vi "Front Grabber Control Read.vi"(1 "Controller State":T1 {"POV" items=["None"=-1, "POV Up"=0, "POV Up Right"=1, "POV Right"=2, "POV Down Right"=3, "POV Down"=4, "POV Down Left"=5, "POV Left"=6, "POV Up Left"=7]}) -> (0 "State out":i16)   [LabVIEW 2010]
uses:
  <vilib>/FTC/FTC ControllerState.ctl
  <vilib>/FTC/FTC POVState.ctl
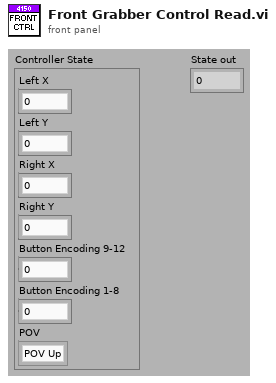
[diagram p1: front panel]
types:
  T1 = typedef "FTC ControllerState.ctl" = cluster{"Left X":i8, "Left Y":i8, "Right X":i8, "Right Y":i8, "Button Encoding 9-12":u8, "Button Encoding 1-8":u8, "POV":T2}
  T2 = typedef "FTC POVState.ctl" = i8
  T3 = typedef "FTC ButtonState.ctl" = cluster{"Button 1":bool, "Button 2":bool, "Button 3":bool, "Button 4":bool, "Button 5":bool, "Button 6":bool, "Button 7":bool, "Button 8":bool, "Button 9":bool, "Button 10":bool, "Button 11":bool, "Button 12":bool, "POV":T2}
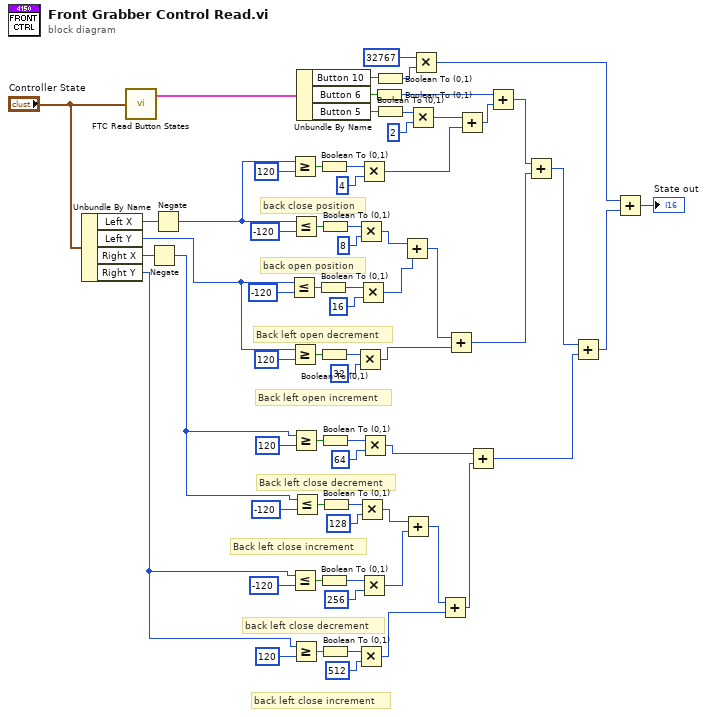
[diagram p0: block diagram]
diagram:
  # "Back left open increment"
  # "Back left open decrement"
  # "back open position"
  # "back left close decrement"
  # "Back left close decrement"
  # "Back left close increment"
  # "back left close increment"
  # "back close position"
  n1 = Unbundle By Name("Controller State") -> ("Left X"=w50:i8, "Left Y"=w40:i8, "Right X"=w14:i8, "Right Y"=w13:i8)
  n2 = call <vilib>:"FTC Read Button States.vi"("Controller State"="Controller State") -> ("Button States"=w53:T3)  [unwired: 2 in, 1 out]
  n3 = Negate(x=w14) -> (-x=w7:i8)
  n4 = Negate(x=w50) -> (-x=w8:i8)
  n5 = Less Or Equal?(x=w40, y=i8 -120) -> (x <= y?=w43:bool)
  n6 = Greater Or Equal?(x=w8, y=i8 120) -> (x >= y?=w55:bool)
  n7 = Greater Or Equal?(x=w40, y=i8 120) -> (x >= y?=w44:bool)
  n8 = Less Or Equal?(x=w13, y=i8 -120) -> (x <= y?=w28:bool)
  n9 = Less Or Equal?(x=w8, y=i8 -120) -> (x <= y?=w56:bool)
  n10 = Greater Or Equal?(x=w7, y=i8 120) -> (x >= y?=w20:bool)
  n11 = Greater Or Equal?(x=w13, y=i8 120) -> (x >= y?=w27:bool)
  n12 = Less Or Equal?(x=w7, y=i8 -120) -> (x <= y?=w19:bool)
  n13 = Unbundle By Name(w53) -> ("Button 10"=w6:bool, "Button 6"=w54:bool, "Button 5"=w63:bool)
  n14 = Boolean To (0,1)(Boolean=w43) -> (0, 1=w45:i16)
  n15 = Boolean To (0,1)(Boolean=w55) -> (0, 1=w57:i16)
  n16 = Boolean To (0,1)(Boolean=w44) -> (0, 1=w47:i16)
  n17 = Boolean To (0,1)(Boolean=w28) -> (0, 1=w26:i16)
  n18 = Boolean To (0,1)(Boolean=w56) -> (0, 1=w61:i16)
  n19 = Boolean To (0,1)(Boolean=w20) -> (0, 1=w18:i16)
  n20 = Boolean To (0,1)(Boolean=w27) -> (0, 1=w24:i16)
  n21 = Boolean To (0,1)(Boolean=w19) -> (0, 1=w16:i16)
  n22 = Multiply(x=w47, y=i16 32) -> (x*y=w36:i16)
  n23 = Multiply(x=w61, y=i16 8) -> (x*y=w39:i16)
  n24 = Multiply(x=w24, y=i16 512) -> (x*y=w34:i16)
  n25 = Multiply(x=w16, y=i16 128) -> (x*y=w31:i16)
  n26 = Multiply(x=w45, y=i16 16) -> (x*y=w38:i16)
  n27 = Multiply(x=w57, y=i16 4) -> (x*y=w68:i16)
  n28 = Multiply(x=w26, y=i16 256) -> (x*y=w32:i16)
  n29 = Multiply(x=w18, y=i16 64) -> (x*y=w12:i16)
  n30 = Boolean To (0,1)(Boolean=w54) -> (0, 1=w58:i16)
  n31 = Boolean To (0,1)(Boolean=w6) -> (0, 1=w5:i16)
  n32 = Boolean To (0,1)(Boolean=w63) -> (0, 1=w64:i16)
  n33 = Add(x=w39, y=w38) -> (x+y=w37:i16)
  n34 = Add(x=w31, y=w32) -> (x+y=w33:i16)
  n35 = Multiply(x=w64, y=i16 2) -> (x*y=w67:i16)
  n36 = Multiply(x=i16 32767, y=w5) -> (x*y=w3:i16)
  n37 = Add(x=w33, y=w34) -> (x+y=w11:i16)
  n38 = Add(x=w37, y=w36) -> (x+y=w35:i16)
  n39 = Add(x=w67, y=w68) -> (x+y=w66:i16)
  n40 = Add(x=w12, y=w11) -> (x+y=w10:i16)
  n41 = Add(x=w58, y=w66) -> (x+y=w59:i16)
  n42 = Add(x=w59, y=w35) -> (x+y=w9:i16)
  n43 = Add(x=w9, y=w10) -> (x+y=w2:i16)
  n44 = Add(x=w3, y=w2) -> (x+y=→"State out":i16)
